vi "Base_posture_reco.vi"(8 "error in (no error)":errorcluster) -> (0 "error out":errorcluster)   [LabVIEW 2017]
uses:
  IP Address.vi
  <vilib>/httpClient/LabVIEWHTTPClient.lvlib
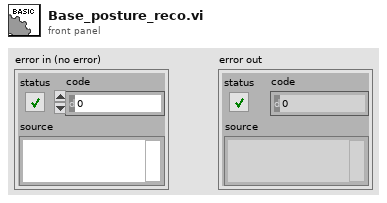
[diagram p1: front panel]
types:
  T1 = enum16{"off", "red", "green", "yellow", "blue", "pink", "cyan", "white"}
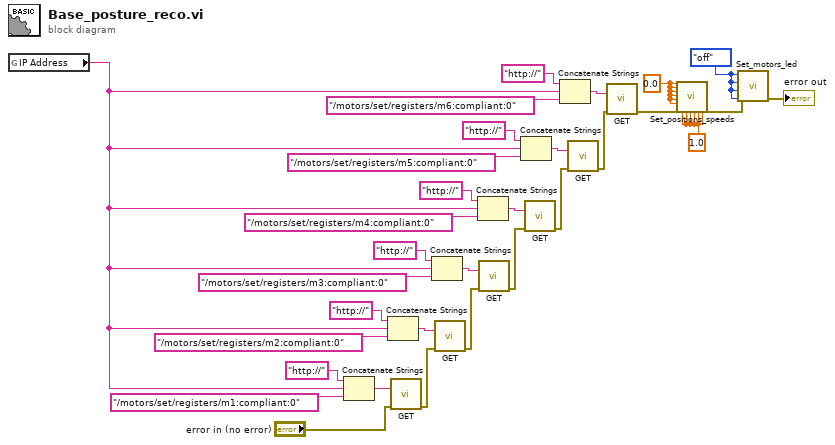
[diagram p0: block diagram]
diagram:
  w28 = T1."off" ("Color m2")
  w31 = 1.0 ("Speed m5")
  w30 = 0.0 ("Speed m5")
  n1 = global read "IP Address.vi" "IP Address"() -> (w1:string)
  n2 = Concatenate Strings("http://" ("string"), w1, "/motors/set/registers/m1:compliant:0" ("string")) -> (w7:string)
  n3 = Concatenate Strings("http://" ("string"), w1, "/motors/set/registers/m2:compliant:0" ("string")) -> (w12:string)
  n4 = call <vilib>:"GET.vi"("url"=w7, "error in (no error)"="error in (no error)") -> ("error out"=w3:errorcluster)  [unwired: 10 in, 3 out]
  n5 = Concatenate Strings("http://" ("string"), w1, "/motors/set/registers/m3:compliant:0" ("string")) -> (w13:string)
  n6 = call <vilib>:"GET.vi"("url"=w12, "error in (no error)"=w3) -> ("error out"=w4:errorcluster)  [unwired: 10 in, 3 out]
  n7 = Concatenate Strings("http://" ("string"), w1, "/motors/set/registers/m4:compliant:0" ("string")) -> (w18:string)
  n8 = call <vilib>:"GET.vi"("url"=w13, "error in (no error)"=w4) -> ("error out"=w5:errorcluster)  [unwired: 10 in, 3 out]
  n9 = Concatenate Strings("http://" ("string"), w1, "/motors/set/registers/m5:compliant:0" ("string")) -> (w20:string)
  n10 = call <vilib>:"GET.vi"("url"=w18, "error in (no error)"=w5) -> ("error out"=w6:errorcluster)  [unwired: 10 in, 3 out]
  n11 = Concatenate Strings("http://" ("string"), w1, "/motors/set/registers/m6:compliant:0" ("string")) -> (w23:string)
  n12 = call <vilib>:"GET.vi"("url"=w20, "error in (no error)"=w6) -> ("error out"=w19:errorcluster)  [unwired: 10 in, 3 out]
  n13 = call <vilib>:"GET.vi"("url"=w23, "error in (no error)"=w19) -> ("error out"=w26:errorcluster)  [unwired: 10 in, 3 out]
  n14 = call "Set_positions_speeds.vi"("m1"=w30, "m2"=w30, "m3"=w30, "m4"=w30, "m5"=w30, "m6"=w30, "error in (no error)"=w26, "Speed m1"=w31, "Speed m2"=w31, "Speed m3"=w31, "Speed m4"=w31, "Speed m5"=w31, "Speed m6"=w31) -> ("error out"=w29:errorcluster)  [unwired: 14 in]
  n15 = call "Set_motors_led.vi"("error in (no error)"=w29, "Color m6"=w28, "Color m5"=w28, "Color m3"=w28, "Color m2"=w28) -> ("error out"=→"error out":errorcluster)  [unwired: 6 in]
